vi "1B_AnalyzePulseTrain_wOptions_Sub.vi"(0 "Filtered data":waveform(dbl), 1 "Repetitions in the Input Waveform":i32, 5 "Offset":dbl, 7 "Pulse Characteristics":T2) -> (4 "Frequency":dbl, 6 "Avg. CBC Amplitude":dbl, 8 "Stim PW":dbl[](array[numeric]), 9 "Recovery Holdoff":dbl[](array[numeric]), 10 "Waveform Parameters":T1, 11 "Recovery Amplitude":dbl[](array[numeric]), 12 "Stim Amplitude":dbl[](array[numeric]), 13 "Avg. CBC Width":dbl, 14 "Recovery PW":dbl[](array[numeric]), 15 "Interphase Delay":dbl[](array[numeric]))   [LabVIEW 2010]
uses:
  <vilib>/measure/mamon.llb/Trigger Detection for 1 Channel.vi
  <vilib>/measure/NI_MAPro.lvlib
  <vilib>/Analysis/NI_AALBase.lvlib
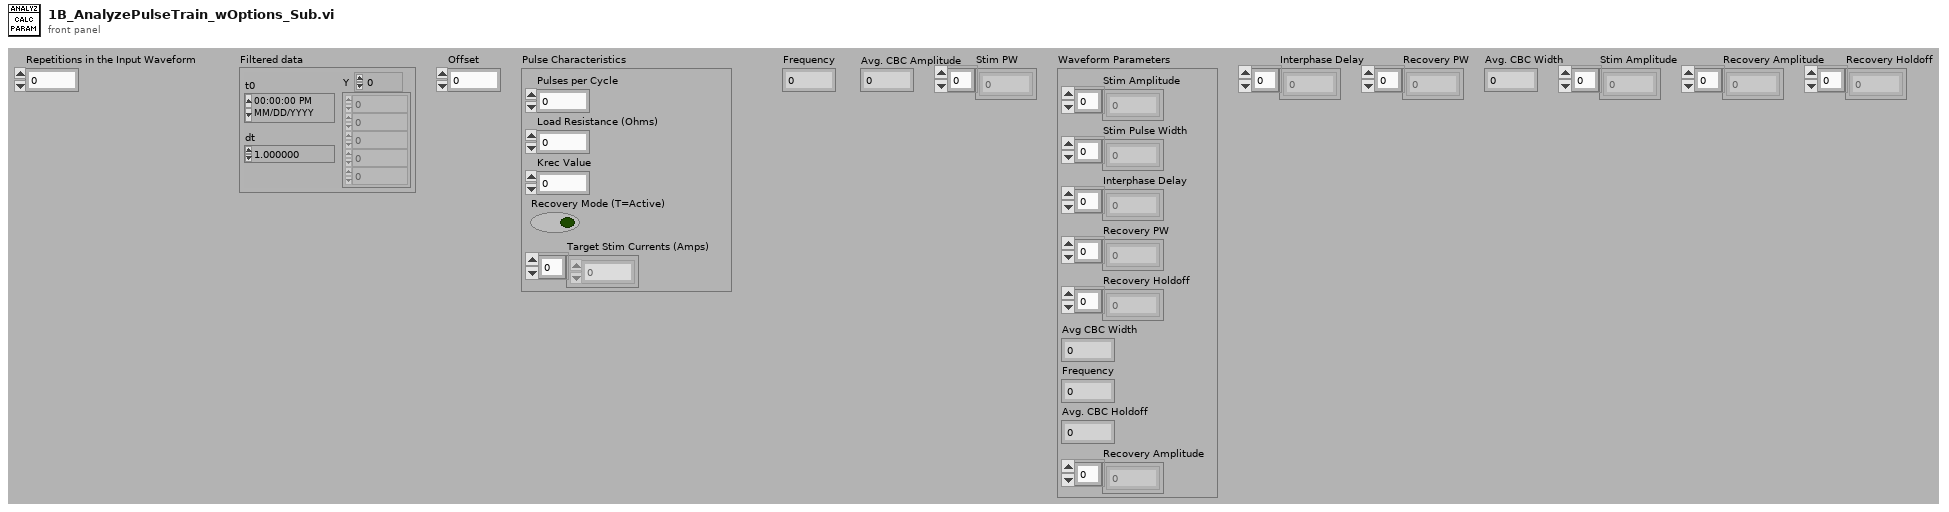
[diagram p1: front panel]
types:
  T1 = cluster{"Stim Amplitude":dbl[], "Stim Pulse Width":dbl[], "Interphase Delay":dbl[], "Recovery PW":dbl[], "Recovery Holdoff":dbl[], "Avg CBC Width":dbl, "Frequency":dbl, "Avg. CBC Holdoff":dbl, "Recovery Amplitude":dbl[]}
  T2 = cluster{"Pulses per Cycle":i32, "Load Resistance (Ohms)":dbl, "Krec Value":i32, "Recovery Mode (T=Active)":bool, "Target Stim Currents (Amps)":dbl[]}
  T3 = cluster{"trigger slope":u16, "Trigger Level":dbl}[]
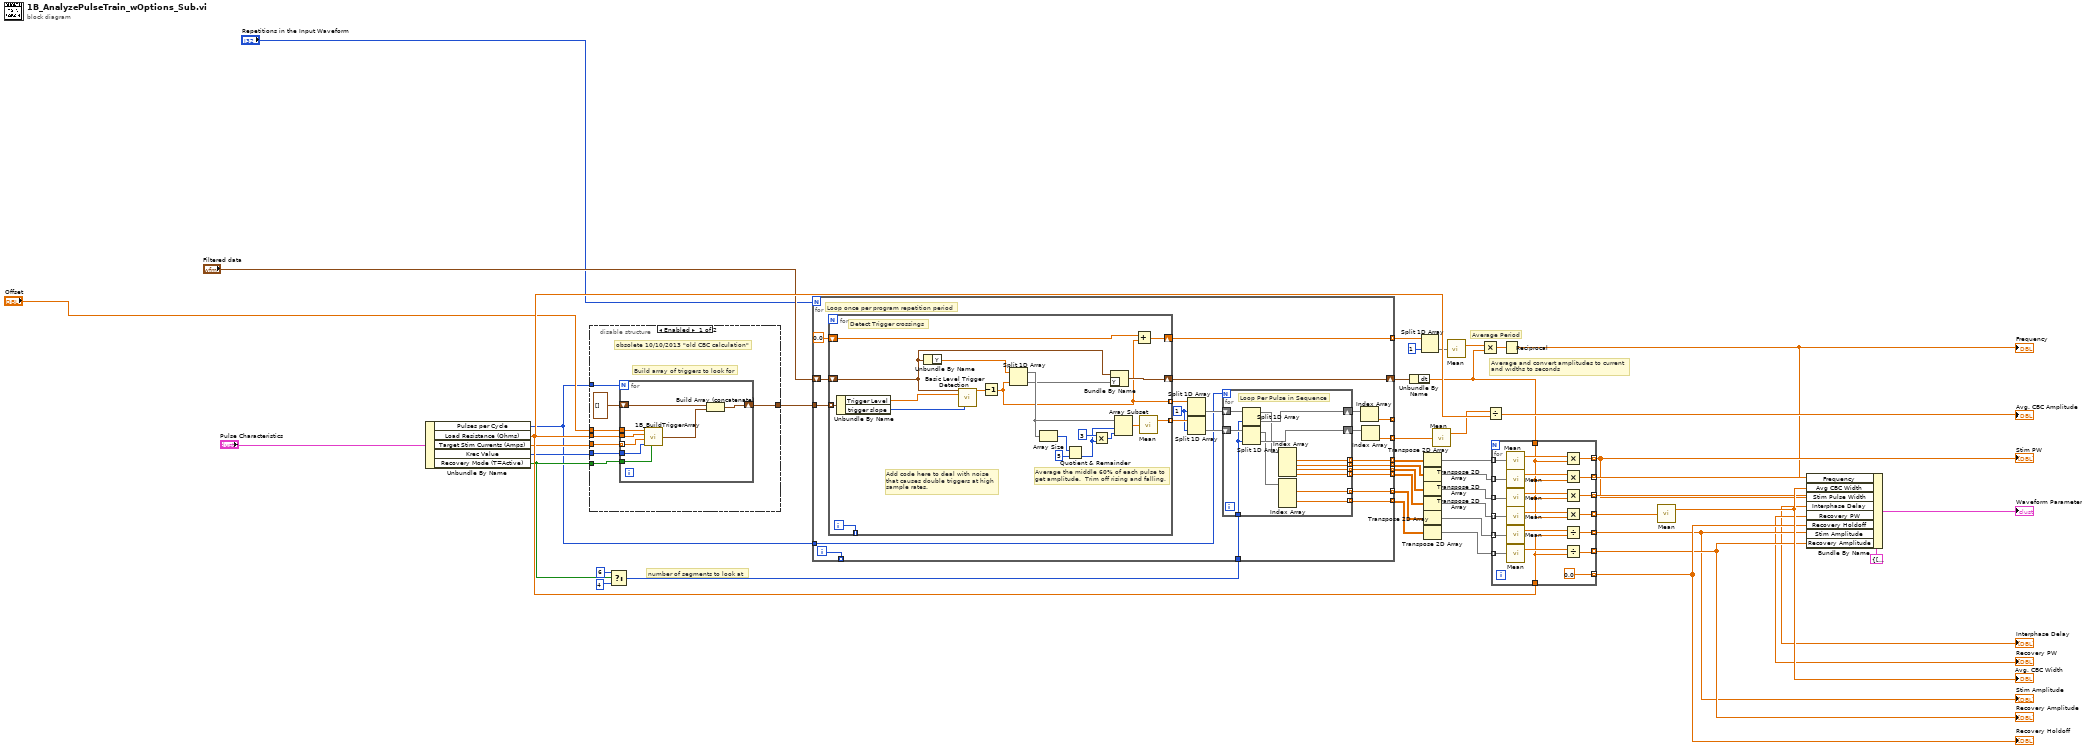
[diagram p0: block diagram]
diagram:
  # "number of segments to look at"
  # "Average Period"
  # "Average and convert amplitudes to current\nand widths to seconds"
  n1 = Unbundle By Name("Pulse Characteristics") -> ("Pulses per Cycle"=w14:i32, "Load Resistance (Ohms)"=w46:dbl, "Target Stim Currents (Amps)"=w42:dbl[], "Krec Value"=w15:i32, "Recovery Mode (T=Active)"=w37:bool)
  n2 = disable-structure shown="Enabled" {
    disable-tunnel: w14 -> [w53 _]
    disable-tunnel: w15 -> [w52 _]
    disable-tunnel: [w51 _] -> w33
    disable-tunnel: w37 -> [w50 _]
    disable-tunnel: w46 -> [w49 _]
    disable-tunnel: w42 -> [w48 _]
    disable-tunnel: "Offset" -> [w47 _]
    frame Enabled {
      # "obsolete 10/10/2013 \"old CBC calculation\""
      # "Build array of triggers to look for"
      n3 = for {
        N: w53 -> [_]
        shift-right: [w62] -> w51
        shift-left: T3 [] -> [w61]
        tunnel: w47 -> [w60]
        tunnel: w50 -> [w59]
        tunnel: w49 -> [w58]
        tunnel: w48 -> [w57] mode=indexing
        tunnel: w52 -> [w56]
        n4 = call "1B_BuildTriggerArray.vi"("CBC Trigger Level"=w60, "Load Resistance (Ohms)"=w58, "Target Stim Current (Amps)"=w57, "Krec Value"=w56, "Recovery Mode (T=Active)"=w59) -> ("Pulse Triggers"=w55:T3)
        n5 = Build Array (concatenate)(w61, w55) -> (w62:T3)
      }
    }
    frame Disabled {
      # "New as of 10/10/2013: New way to calculate CBC on\nlast pulse only"
    }
  }
  n6 = Select(t=6, s=w37, f=4 ("index")) -> (s? t:f=w39:i32)
  n7 = for {
    N: "Repetitions in the Input Waveform" -> [_]
    tunnel: w33 -> [w85]
    shift-right: [w81] -> w17
    shift-left: "Filtered data" -> [w84]
    tunnel: w14 -> [w78]
    tunnel: [w75] -> _ mode=indexing
    tunnel: [w74] -> w1 mode=indexing
    tunnel: [w73] -> w2 mode=indexing
    tunnel: [w72] -> w3 mode=indexing
    tunnel: [w71] -> w4 mode=indexing
    tunnel: [w70] -> w5 mode=indexing
    tunnel: [w69] -> w6 mode=indexing
    tunnel: [w68] -> w7 mode=indexing
    tunnel: [w65] -> w19 mode=indexing
    tunnel: w39 -> [w64]
    tunnel: [w63] -> _ mode=indexing
    i -> [w63]
    w82 = 1 ("index")
    # "Loop once per program repetition period"
    n8 = for {
      tunnel: w85 -> [w118] mode=indexing
      shift-right: [w106] -> w81
      shift-left: w84 -> [w102]
      tunnel: [w110] -> w83 mode=indexing
      tunnel: [w104] -> w66 mode=indexing
      shift-right: [w109] -> w65
      shift-left: 0.0 -> [w108]
      tunnel: [w99] -> _ mode=indexing
      i -> [w99]
      # "Add code here to deal with noise \nthat causes double triggers at high\nsample rates."
      # "Detect Trigger crossings"
      # "Average the middle 60% of each pulse to\nget amplitude.  Trim off rising and falling."
      n9 = Unbundle By Name(w118) -> ("Trigger Level"=w100:dbl, "trigger slope"=w107:u16)
      n10 = Unbundle By Name(w102) -> ("Y"=w103:dbl[])
      n11 = call-poly <vilib>:"Basic Level Trigger Detection.vi"("signal in"=w102, "level"=w100, "trigger slope"=w107) -> ("trigger location"=w101:dbl)  [unwired: 10 in, 2 out]
      n12 = Decrement(x=w101) -> (x-1=w104:dbl)
      n13 = Split 1D Array(array=w103, index=w104) -> (first subarray=w112:dbl[], second subarray=w105:dbl[])
      n14 = Array Size(array=w112) -> (size(s)=w117:i32)
      n15 = Quotient & Remainder(x=w117, y=5) -> (floor(x/y)=w114:i32)  [unwired: 1 out]
      n16 = Multiply(x=3, y=w114) -> (x*y=w113:i32)
      n17 = Bundle By Name(cluster=w102, "Y"=w105) -> (w106:waveform(dbl))
      n18 = Array Subset(array=w112, index=w114, length=w113) -> (w111:dbl[])
      n19 = Add(x=w108, y=w104) -> (x+y=w109:dbl)
      n20 = call <vilib>:"Mean.vi"("X"=w111) -> ("mean"=w110:dbl)  [unwired: 1 out]
    }
    n21 = Split 1D Array(array=w66, index=w82) -> (second subarray=w80:dbl[])  [unwired: 1 out]
    n22 = Split 1D Array(array=w83, index=w82) -> (second subarray=w79:dbl[])  [unwired: 1 out]
    n23 = for {
      N: w78 -> [_]
      shift-right: [w96] -> w77
      shift-left: w80 -> [w98]
      shift-right: [w95] -> w76
      shift-left: w79 -> [w97]
      tunnel: [w92] -> w73 mode=indexing
      tunnel: [w91] -> w72 mode=indexing
      tunnel: [w90] -> w71 mode=indexing
      tunnel: [w89] -> w70 mode=indexing
      tunnel: [w88] -> w69 mode=indexing
      tunnel: [w87] -> w68 mode=indexing
      tunnel: w64 -> [w86]
      # "Loop Per Pulse in Sequence"
      n24 = Split 1D Array(array=w98, index=w86) -> (first subarray=w94:dbl[], second subarray=w96:dbl[])
      n25 = Split 1D Array(array=w97, index=w86) -> (first subarray=w93:dbl[], second subarray=w95:dbl[])
      n26 = Index Array(array=w94) -> (element #1=w92:dbl, element #2=w91:dbl, element #3=w90:dbl, element #4=w89:dbl)  [unwired: 4 in]
      n27 = Index Array(array=w93) -> (element #1=w88:dbl, element #3=w87:dbl)  [unwired: 4 in, 2 out]
    }
    n28 = Index Array(array=w77) -> (element=w75:dbl)  [unwired: 1 in]
    n29 = Index Array(array=w76) -> (element=w74:dbl)  [unwired: 1 in]
  }
  n30 = Unbundle By Name(w17) -> ("dt"=w22:dbl)
  n31 = Split 1D Array(array=w19, index=1) -> (second subarray=w20:dbl[])  [unwired: 1 out]
  n32 = Transpose 2D Array(2D array=w2) -> (transposed array=w8:dbl[][])
  n33 = Transpose 2D Array(2D array=w3) -> (transposed array=w9:dbl[][])
  n34 = Transpose 2D Array(2D array=w4) -> (transposed array=w10:dbl[][])
  n35 = Transpose 2D Array(2D array=w5) -> (transposed array=w11:dbl[][])
  n36 = Transpose 2D Array(2D array=w6) -> (transposed array=w12:dbl[][])
  n37 = Transpose 2D Array(2D array=w7) -> (transposed array=w13:dbl[][])
  n38 = call <vilib>:"Mean.vi"("X"=w1) -> ("mean"=w18:dbl)  [unwired: 1 out]
  n39 = call <vilib>:"Mean.vi"("X"=w20) -> ("mean"=w21:dbl)  [unwired: 1 out]
  n40 = Multiply(x=w21, y=w22) -> (x*y=w23:dbl)
  n41 = Divide(x=w18, y=w46) -> (x/y=→"Avg. CBC Amplitude":dbl)
  n42 = for {
    tunnel: w8 -> [w139] mode=indexing
    tunnel: w9 -> [w138] mode=indexing
    tunnel: w10 -> [w137] mode=indexing
    tunnel: w11 -> [w136] mode=indexing
    tunnel: w12 -> [w135] mode=indexing
    tunnel: w13 -> [w134] mode=indexing
    tunnel: [w133] -> w28 mode=indexing
    tunnel: [w132] -> w29 mode=indexing
    tunnel: [w131] -> w30 mode=indexing
    tunnel: [w130] -> w35 mode=indexing
    tunnel: [w129] -> w31 mode=indexing
    tunnel: [w128] -> w32 mode=indexing
    tunnel: w22 -> [w121]
    tunnel: w46 -> [w120]
    tunnel: [0.0 ("Load Resistance (Ohms)")] -> w34 mode=indexing
    n43 = call <vilib>:"Mean.vi"("X"=w139) -> ("mean"=w126:dbl)  [unwired: 1 out]
    n44 = call <vilib>:"Mean.vi"("X"=w138) -> ("mean"=w125:dbl)  [unwired: 1 out]
    n45 = call <vilib>:"Mean.vi"("X"=w137) -> ("mean"=w124:dbl)  [unwired: 1 out]
    n46 = call <vilib>:"Mean.vi"("X"=w136) -> ("mean"=w123:dbl)  [unwired: 1 out]
    n47 = call <vilib>:"Mean.vi"("X"=w135) -> ("mean"=w122:dbl)  [unwired: 1 out]
    n48 = call <vilib>:"Mean.vi"("X"=w134) -> ("mean"=w127:dbl)  [unwired: 1 out]
    n49 = Multiply(x=w126, y=w121) -> (x*y=w133:dbl)
    n50 = Multiply(x=w125, y=w121) -> (x*y=w132:dbl)
    n51 = Multiply(x=w124, y=w121) -> (x*y=w131:dbl)
    n52 = Multiply(x=w123, y=w121) -> (x*y=w130:dbl)
    n53 = Divide(x=w122, y=w120) -> (x/y=w129:dbl)
    n54 = Divide(x=w127, y=w120) -> (x/y=w128:dbl)
  }
  "Recovery Holdoff" <- w34
  "Recovery Amplitude" <- w32
  "Stim Amplitude" <- w31
  "Recovery PW" <- w30
  "Interphase Delay" <- w29
  "Stim PW" <- w28
  n55 = Reciprocal(x=w23) -> (1/x=w26:dbl)
  "Frequency" <- w26
  n56 = call <vilib>:"Mean.vi"("X"=w35) -> ("mean"=w36:dbl)  [unwired: 1 out]
  "Avg. CBC Width" <- w36
  n57 = Bundle By Name(cluster=T1 {"Stim Amplitude"=[], "Stim Pulse Width"=[], "Interphase Delay"=[], "Recovery PW"=[], "Recovery Holdoff"=[], "Avg CBC Width"=0.0, "Frequency"=0.0, "Avg. CBC Holdoff"=0.0, "Recovery Amplitude"=[]} ("Pulse Train Parameters"), "Frequency"=w26, "Avg CBC Width"=w36, "Stim Pulse Width"=w28, "Interphase Delay"=w29, "Recovery PW"=w30, "Recovery Holdoff"=w34, "Stim Amplitude"=w31, "Recovery Amplitude"=w32) -> (→"Waveform Parameters":T1)
